vi "Read Script.vi"(2 "commands":string, 3 "script name":string) -> (0 "text from file":string, 1 "output array":dbl[][](array[numeric]))   [LabVIEW 2014]
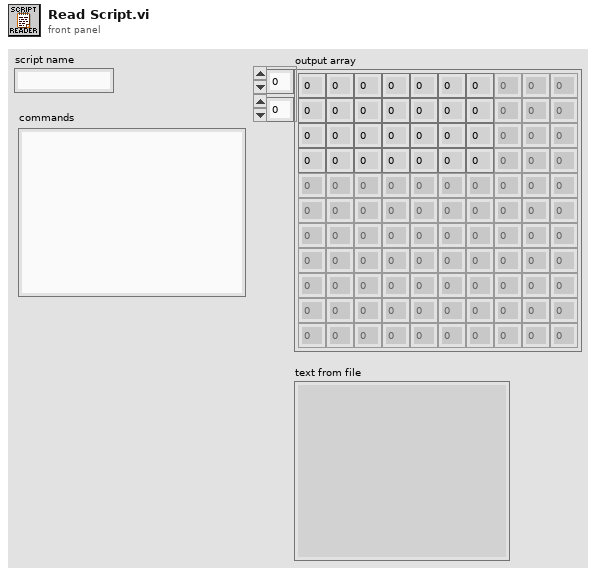
[diagram p1: front panel]
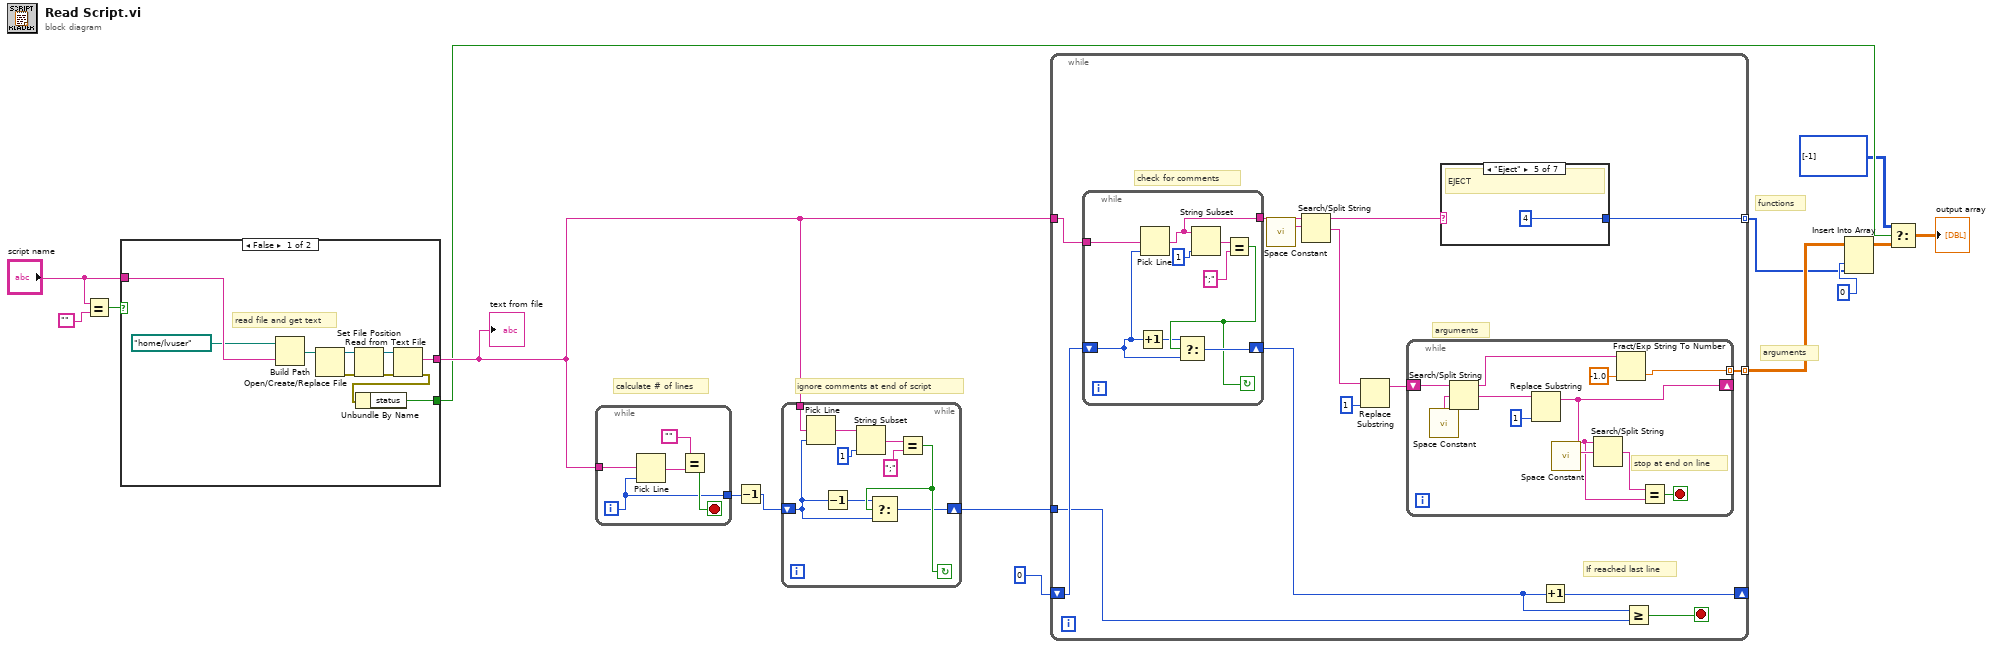
[diagram p0: block diagram]
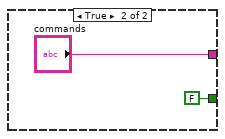
[diagram p2: hidden frame]
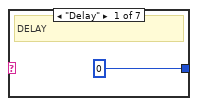
[diagram p3: hidden frame]
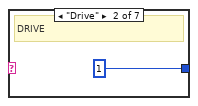
[diagram p4: hidden frame]
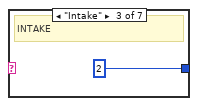
[diagram p5: hidden frame]
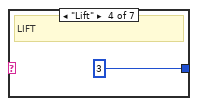
[diagram p6: hidden frame]
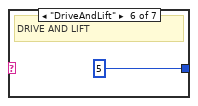
[diagram p7: hidden frame]
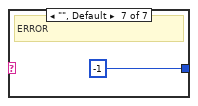
[diagram p8: hidden frame]
diagram:
  # "ignore comments at end of script"
  # "calculate # of lines"
  # "arguments"
  # "functions"
  n1 = Equal?(x="script name", y="") -> (x = y?=w6:bool)
  n2 = case shown="False" w6 {
    tunnel: "script name" -> [w22 _]
    tunnel: [w21 "commands"] -> w12
    tunnel: [w18 FALSE ("status")] -> w3
    frame False {
      # "read file and get text"
      n3 = Build Path(base path=path "/home/lvuser" ("configuration file path"), name or relative path=w22) -> (appended path=w23:path)
      n4 = Open/Create/Replace File(file path (use dialog)=w23) -> (refnum out=w25:refnum<file>, error out=w19:errorcluster)  [unwired: 5 in, 1 out]
      n5 = Set File Position(refnum=w25, error in=w19) -> (refnum out=w24:refnum<file>, error out=w20:errorcluster)  [unwired: 2 in]
      n6 = Read from Text File(file (use dialog)=w24, error in=w20) -> (text=w21:string, error out=w17:errorcluster)  [unwired: 2 in, 2 out]
      n7 = Unbundle By Name(w17) -> ("status"=w18:bool)
    }
    frame True {
    }
  }
  "text from file" <- w12
  n8 = while {
    tunnel: w12 -> [w32]
    tunnel: [w28] -> w10
    i -> [w28]
    stop <- w29 stop-if-true
    n9 = Pick Line(multi-line string=w32, line index=w28) -> (output string=w31:string)  [unwired: 1 in]
    n10 = Equal?(x="", y=w31) -> (x = y?=w29:bool)
  }
  n11 = Decrement(x=w10) -> (x-1=w9:i32)
  n12 = while {
    tunnel: w12 -> [w41]
    shift-right: [w34] -> w11
    shift-left: w9 -> [w33]
    stop <- w36 continue-if-true
    n13 = Pick Line(multi-line string=w41, line index=w33) -> (output string=w39:string)  [unwired: 1 in]
    n14 = Decrement(x=w33) -> (x-1=w35:i32)
    n15 = String Subset(string=w39, length (rest)=1 ("length (rest)")) -> (substring=w38:string)  [unwired: 1 in]
    n16 = Equal?(x=w38, y=";") -> (x = y?=w36:bool)
    n17 = Select(t=w35, s=w36, f=w33) -> (s? t:f=w34:i32)
  }
  n18 = while {
    tunnel: w12 -> [w48]
    tunnel: [w54] -> w14 mode=indexing
    shift-right: [w45] -> _
    shift-left: 0 -> [w50]
    tunnel: w11 -> [w46]
    tunnel: [w42] -> w1 mode=indexing
    stop <- w47 stop-if-true
    # "arguments"
    # "If reached last line"
    # "check for comments"
    n19 = while {
      tunnel: w48 -> [w71]
      tunnel: [w67] -> w49
      shift-right: [w66] -> w44
      shift-left: w50 -> [w63]
      stop <- w65 continue-if-true
      n20 = Increment(x=w63) -> (x+1=w64:i32)
      n21 = Pick Line(multi-line string=w71, line index=w63) -> (output string=w67:string)  [unwired: 1 in]
      n22 = String Subset(string=w67, length (rest)=1 ("length (rest)")) -> (substring=w69:string)  [unwired: 1 in]
      n23 = Equal?(x=w69, y=";") -> (x = y?=w65:bool)
      n24 = Select(t=w64, s=w65, f=w63) -> (s? t:f=w66:i32)
    }
    n25 = call <vilib>:"Space Constant.vi"() -> ("String"=w55:string)
    n26 = Search/Split String(string=w49, search string/char (-)=w55) -> (substring before match=w43:string, match + rest of string=w53:string)  [unwired: 1 in, 1 out]
    n27 = Replace Substring(2:1 ("length (len. of substring)"), 5:w53) -> (1:w51:string)  [unwired: 2 in, 1 out]
    n28 = while {
      shift-right: [w73] -> _
      shift-left: w51 -> [w74]
      tunnel: [w77] -> w54 mode=indexing
      stop <- w81 stop-if-true
      # "stop at end on line"
      n29 = call <vilib>:"Space Constant.vi"() -> ("String"=w82:string)
      n30 = Search/Split String(string=w74, search string/char (-)=w82) -> (substring before match=w78:string, match + rest of string=w80:string)  [unwired: 1 in, 1 out]
      n31 = Replace Substring(2:1 ("length (len. of substring)"), 5:w80) -> (1:w73:string)  [unwired: 2 in, 1 out]
      n32 = call <vilib>:"Space Constant.vi"() -> ("String"=w76:string)
      n33 = Search/Split String(string=w73, search string/char (-)=w76) -> (match + rest of string=w75:string)  [unwired: 1 in, 2 out]
      n34 = Fract/Exp String To Number(string=w78, default (0 dbl)=-1.0 ("default (0 DBL)")) -> (number=w77:dbl)  [unwired: 2 in, 1 out]
      n35 = Equal?(x=w75, y=w73) -> (x = y?=w81:bool)
    }
    n36 = case shown="\"Eject\"" w43 {
      tunnel: [0 1 2 3 4 5 -1] -> w42
      frame "Delay" {
        # "DELAY"
      }
      frame "Drive" {
        # "DRIVE"
      }
      frame "Intake" {
        # "INTAKE"
      }
      frame "Lift" {
        # "LIFT"
      }
      frame "Eject" {
        # "EJECT"
      }
      frame "DriveAndLift" {
        # "DRIVE AND LIFT"
      }
      frame "", Default {
        # "ERROR"
      }
    }
    n37 = Increment(x=w44) -> (x+1=w45:i32)
    n38 = Greater Or Equal?(x=w44, y=w46) -> (x >= y?=w47:bool)
  }
  n39 = Insert Into Array(array=w14, index (col)=0 ("disabled index (col)"), new element=w1) -> (w4:dbl[][])  [unwired: 1 in]
  n40 = Select(t=i32[][] [[-1]], s=w3, f=w4) -> (s? t:f=→"output array":dbl[][])
